vi "State_Machine.vi"(8 "error in (no error)":errorcluster caption="entrée d'erreur (pas d'erreur)", 11 "Delay en entrée":refnum<class "Enter_ID_Enocean.lvclass">) -> (0 "error out":errorcluster caption="sortie d'erreur", 2 "Json_String":string, 3 "Delay en sortie":refnum<class "Enter_ID_Enocean.lvclass">)   [LabVIEW 2020, in "Library Test.lvlib" / "Enter_ID_Enocean.lvclass"]
uses:
  Enter_ID_Enocean.lvclass
  C:/Users/ngarcin/OneDrive - Altyor/Standard TB/Suite TB45/Class/Test/Test (Default)/Test (Default).lvclass
  Popup/Class Popup Operator_Input EMS_Code/Class Popup Operator_Input EMS_Code.lvclass
  C:/Users/ngarcin/OneDrive - Altyor/Standard TB/Suite TB45/Class/Popup/Class Popup (Main)/Class Popup (Main).lvclass
  Commun VI/TypeDef/Variable Printable.ctl
  JSON API/Variant JSON/Variant JSON.lvlib
  JSON API/Get Polymorphic/JSON GetSet.lvlib
  JSON API/JSON Value/Set from JSON string.vi
  JSON API/JSON Value/JSON Value.lvclass
  Commun VI/Library Commun.lvlib
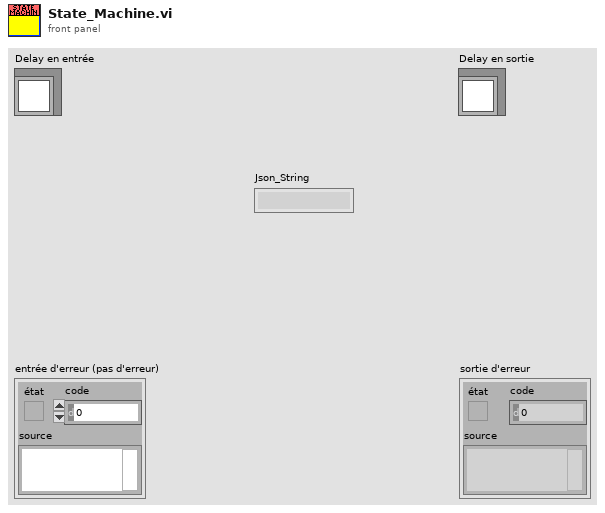
[diagram p1: front panel]
types:
  T1 = typedef "Variable Printable.ctl" = string
  T2 = enum16{"Get Variable", "Get All Variables", "Set Variable", "Delete Variable", "Delete All Variable"}
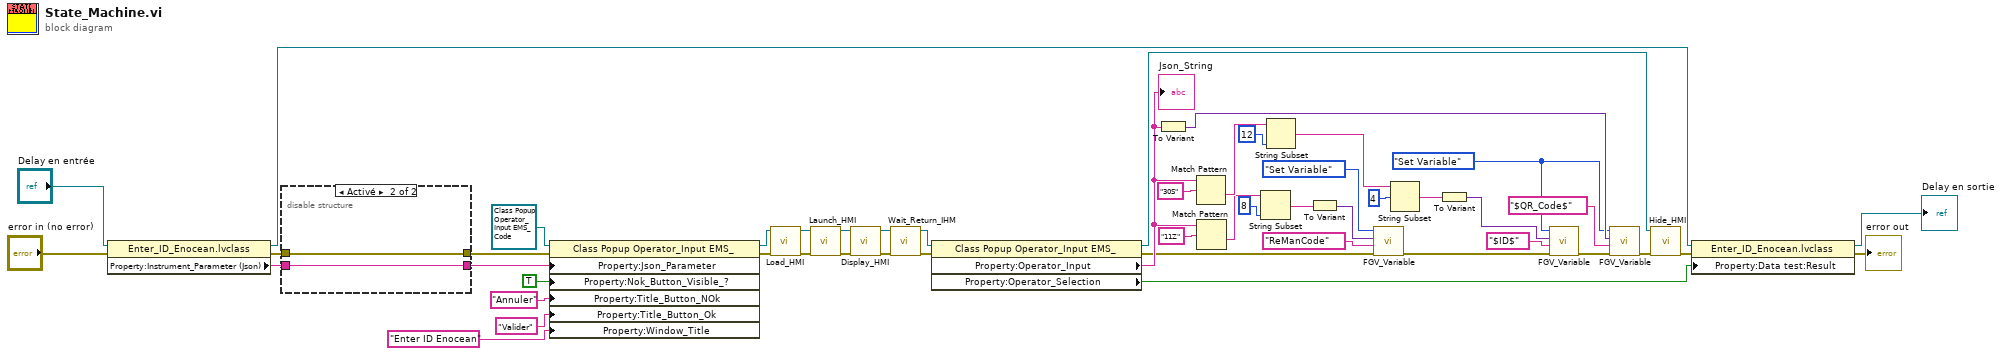
[diagram p0: block diagram]
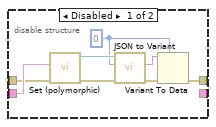
[diagram p2: hidden frame]
diagram:
  w11 = T2."Set Variable" ("Function")
  n1 = property class="Enter_ID_Enocean.lvclass"(reference="Delay en entrée", error in="error in (no error)") -> (reference out=w28:refnum<class "Enter_ID_Enocean.lvclass">, error out=w47:errorcluster, "Property:Instrument_Parameter (Json)"=w49:string)
  n2 = disable-structure shown="Activé" {
    disable-tunnel: w49 -> [w53 w59]
    disable-tunnel: w47 -> [w52 w60]
    disable-tunnel: [w51 w60] -> w34
    disable-tunnel: [_ w59] -> w30
    frame Disabled {
      w54 = u32 0 ("Channel")
      n3 = call-poly "Set (polymorphic).vi"("error in (no error)"=w52, "JSON stream"=w53) -> ("error out"=w56:errorcluster, "JSON Value out"=w58:refnum<class "JSON Value.lvclass">)  [unwired: 7 in, 1 out]
      n4 = call "JSON to Variant.vi"("error in (no error)"=w56, "Variant (Data Type)"=w54, "JSON Value"=w58) -> ("error out"=w57:errorcluster, "Variant out"=w55:variant)  [unwired: 7 in]
      n5 = Variant To Data(error in=w57, type=w54, Variant=w55) -> (error out=w51:errorcluster)  [unwired: 1 out]
    }
    frame Enabled {
    }
  }
  n6 = property class="Class Popup Operator_Input EMS_"(reference=refnum<class "Class Popup Operator_Input EMS_Code.lvclass"> refnum ("Library Popup.lvlib:Class Popup Operator_Input EMS_Code.lvclass"), error in=w34, "Property:Json_Parameter"=w30, "Property:Nok_Button_Visible_?"=TRUE ("Nok_Button_Visible_?"), "Property:Title_Button_NOk"="Annuler" ("Title_Button_NOk"), "Property:Title_Button_Ok"="Valider" ("Title_Button_Ok"), "Property:Window_Title"="Enter ID Enocean" ("Window_Title")) -> (reference out=w40:refnum<class "Class Popup Operator_Input EMS_Code.lvclass">, error out=w39:errorcluster)
  n7 = call-dynamic "Load_HMI.vi"("error in (no error)"=w39, "Class Popup (Default) en entrée"=w40) -> ("error out"=w46:errorcluster, "Class Popup (Default) en sortie"=w45:refnum<class "Class Popup Operator_Input EMS_Code.lvclass">)  [unwired: 8 in]
  n8 = call-dynamic "Launch_HMI.vi"("error in (no error)"=w46, "Class Popup (Default) en entrée"=w45) -> ("error out"=w44:errorcluster, "Class Popup (Default) en sortie"=w42:refnum<class "Class Popup Operator_Input EMS_Code.lvclass">)  [unwired: 8 in]
  n9 = call-dynamic "Display_HMI.vi"("error in (no error)"=w44, "Class Popup (Default) en entrée"=w42) -> ("error out"=w43:errorcluster, "Class Popup (Default) en sortie"=w41:refnum<class "Class Popup Operator_Input EMS_Code.lvclass">)  [unwired: 8 in]
  n10 = call-dynamic "Wait_Return_IHM.vi"("error in (no error)"=w43, "Class Popup (Default) en entrée"=w41) -> ("error out"=w35:errorcluster, "Class Popup (Default) en sortie"=w36:refnum<class "Class Popup Operator_Input EMS_Code.lvclass">)  [unwired: 8 in]
  n11 = property class="Class Popup Operator_Input EMS_"(reference=w36, error in=w35) -> (reference out=w29:refnum<class "Class Popup Operator_Input EMS_Code.lvclass">, error out=w2:errorcluster, "Property:Operator_Input"=w7:string, "Property:Operator_Selection"=w26:bool)
  "Json_String" <- w7
  n12 = To Variant(anything=w7) -> (Variant=w12:variant)
  n13 = Match Pattern(string=w7, regular expression="30S" ("chaîne")) -> (after substring=w18:string)  [unwired: 1 in, 3 out]
  n14 = Match Pattern(string=w7, regular expression="11Z" ("chaîne")) -> (after substring=w5:string)  [unwired: 1 in, 3 out]
  n15 = String Subset(string=w5, length (rest)=8 ("longueur (reste)")) -> (substring=w4:string)  [unwired: 1 in]
  n16 = String Subset(string=w18, length (rest)=12 ("longueur (reste)")) -> (substring=w20:string)  [unwired: 1 in]
  n17 = To Variant(anything=w4) -> (Variant=w3:variant)
  n18 = call "FGV_Variable.vi"("error in (no error)"=w2, "Variable"=T1 "ReManCode", "Data In"=w3, "Function"=T2."Set Variable") -> ("error out"=w1:errorcluster)  [unwired: 5 in, 2 out]
  n19 = String Subset(string=w20, offset (0)=4) -> (substring=w17:string)  [unwired: 1 in]
  n20 = To Variant(anything=w17) -> (Variant=w16:variant)
  n21 = call "FGV_Variable.vi"("error in (no error)"=w1, "Variable"=T1 "$ID$", "Data In"=w16, "Function"=w11) -> ("error out"=w14:errorcluster)  [unwired: 5 in, 2 out]
  n22 = call "FGV_Variable.vi"("error in (no error)"=w14, "Variable"=T1 "$QR_Code$", "Data In"=w12, "Function"=w11) -> ("error out"=w13:errorcluster)  [unwired: 5 in, 2 out]
  n23 = call-dynamic "Hide_HMI.vi"("error in (no error)"=w13, "Class Popup (Default) en entrée"=w29) -> ("error out"=w27:errorcluster)  [unwired: 8 in, 1 out]
  n24 = property class="Enter_ID_Enocean.lvclass"(reference=w28, error in=w27, "Property:Data test:Result"=w26) -> (reference out=→"Delay en sortie":refnum<class "Enter_ID_Enocean.lvclass">, error out=→"error out":errorcluster)
